vi "AM modulation_test.vi"() -> ()   [LabVIEW 2017]
uses:
  <vilib>/Analysis/baseanly.llb/Unit Vector (DBL).vi
  <vilib>/Analysis/3filter.llb/FIR Filter (DBL).vi
  <vilib>/Analysis/NI_AALBase.lvlib
  <vilib>/Analysis/NI_AALPro.lvlib
panel:
  out "ASK Modulation signal + Noise":waveform(dbl)(graph)
  out "ASK Modulation signal + Noise":waveform(dbl)(graph)
  in  "SNR(dB)":dbl=6.0
  out "불리언":bool
  out "ASK Modulation signal3":waveform(dbl)(graph)
  out "ASK Modulation signal 2":waveform(dbl)(graph)
  out "크기 2":i32
  in  "Carrier Frequency(Hz)":dbl=50000.0
  out "ASK Modulation signal":waveform(dbl)(graph)
  in  "ID":string="0110"
  out "Data Array 1":dbl[](array[numeric])
  out "Data Array 0":dbl[](array[numeric])
  in  "Data(1) time(sec)":dbl=0.1
  in  "Frequency(Hz)":dbl=30000.0
  in  "Amplitude(Vpeak)":dbl=1.0
  in  "Sampling frequency(Hz)":dbl=100000.0
  in  "Data(0) time(sec)":dbl=0.1
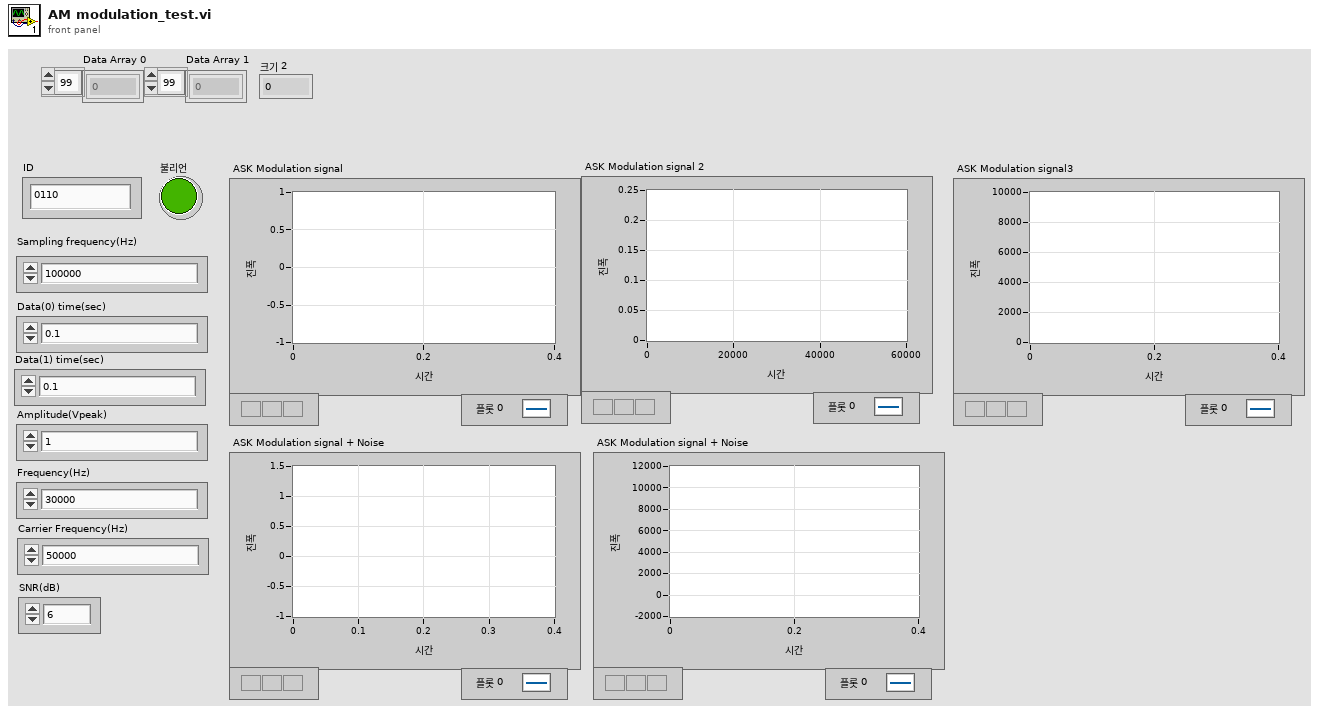
[diagram p1: front panel]
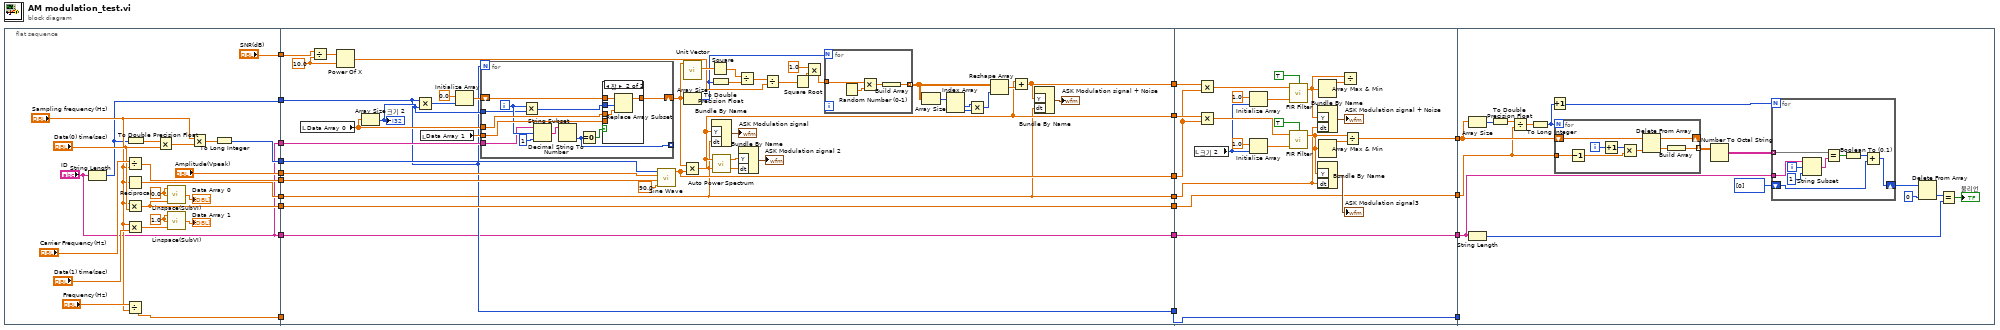
[diagram p0: block diagram]
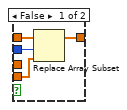
[diagram p2: hidden frame]
diagram:
  n1 = flat-sequence {
    tunnel: [w36] -> w21
    tunnel: ["Amplitude(Vpeak)"] -> w20
    tunnel: [w33] -> w19
    tunnel: [w32] -> w18
    tunnel: ["ID"] -> w17
    tunnel: [w24] -> w16
    tunnel: [w26] -> w12
    tunnel: [w25] -> w11
    tunnel: ["ID"] -> w5
    tunnel: ["SNR(dB)"] -> w2
    tunnel: w21 -> [w78]
    tunnel: w20 -> [w76]
    tunnel: w19 -> [_]
    tunnel: w18 -> [w49]
    tunnel: w17 -> [w77]
    tunnel: w16 -> [w69]
    tunnel: [w50] -> w15
    tunnel: [w72] -> w14
    tunnel: [w49] -> w13
    tunnel: w12 -> [w71]
    tunnel: w11 -> [w70]
    tunnel: [w70] -> w10
    tunnel: [w69] -> w6
    tunnel: w5 -> [w68]
    tunnel: [w68] -> w3
    tunnel: w2 -> [w67]
    tunnel: [w47] -> w1
    tunnel: w15 -> [w133]
    tunnel: w14 -> [w113]
    tunnel: w13 -> [w111]
    tunnel: w10 -> [w127]
    tunnel: [w124] -> w9
    tunnel: [w127] -> w8
    tunnel: [w123] -> w7
    tunnel: w6 -> [w123]
    tunnel: [w122] -> w4
    tunnel: w3 -> [w122]
    tunnel: w1 -> [w112]
    tunnel: w9 -> [w146]
    tunnel: w8 -> [w145]
    tunnel: w7 -> [_]
    tunnel: w4 -> [w139]
    frame #0 {
      w41 = 1.0 ("Start")
      w43 = 0.0 ("Start")
      n2 = String Length(string="ID") -> (length=w24:i32)
      n3 = Divide(x="Carrier Frequency(Hz)", y="Sampling frequency(Hz)") -> (x/y=w26:dbl)
      n4 = Reciprocal(x="Sampling frequency(Hz)") -> (1/x=w32:dbl)
      n5 = Multiply(x="Sampling frequency(Hz)", y="Data(0) time(sec)") -> (x*y=w25:dbl)
      n6 = Multiply(x="Sampling frequency(Hz)", y="Data(1) time(sec)") -> (x*y=w40:dbl)
      n7 = Divide(x="Frequency(Hz)", y="Sampling frequency(Hz)") -> (x/y=w33:dbl)
      n8 = To Double Precision Float(number=w24) -> (double precision float=w30:dbl)
      n9 = Multiply(x=w30, y="Data(0) time(sec)") -> (x*y=w29:dbl)
      n10 = call "Linspace(SubVI).vi"("NumElements"=w25, "End"=w43, "Start"=w43) -> ("Array"=→"Data Array 0":dbl[])
      n11 = call "Linspace(SubVI).vi"("NumElements"=w40, "End"=w41, "Start"=w41) -> ("Array"=→"Data Array 1":dbl[])
      n12 = Multiply(x="Sampling frequency(Hz)", y=w29) -> (x*y=w37:dbl)
      n13 = To Long Integer(number=w37) -> (32bit integer=w36:i32)
    }
    frame #1 {
      w66 = 10.0 ("y")
      n14 = local read "Data Array 0"() -> (w84:dbl[])
      n15 = Divide(x=w67, y=w66) -> (x/y=w65:dbl)
      n16 = Power Of X(1:w66, 2:w65) -> (0:w59:dbl)
      n17 = Array Size(array=w84) -> (size(s)=w82:i32)
      "크기 2" <- w82
      n18 = Multiply(x=w69, y=w82) -> (x*y=w83:i32)
      n19 = local read "Data Array 1"() -> (w86:dbl[])
      n20 = Initialize Array(0.0 ("원소"), w83) -> (w81:dbl[])
      n21 = for {
        N: w69 -> [_]
        tunnel: w84 -> [w99]
        tunnel: w86 -> [w98]
        shift-right: [w96] -> w63
        shift-left: w81 -> [w97]
        tunnel: w82 -> [w94]
        tunnel: [w92] -> _ mode=indexing
        tunnel: w77 -> [w91]
        i -> [w95]
        n22 = Multiply(x=w95, y=w94) -> (x*y=w93:i32)
        n23 = String Subset(string=w91, offset (0)=w95, length (rest)=1 ("길이(나머지)")) -> (substring=w101:string)
        n24 = Decimal String To Number(string=w101) -> (number=w92:i32)  [unwired: 2 in, 1 out]
        n25 = Equal To 0?(x=w92) -> (x = 0?=w100:bool)
        n26 = case shown="참" w100 {
          tunnel: w99 -> [_ w107]
          tunnel: w98 -> [w103 _]
          tunnel: w97 -> [w106 w110]
          tunnel: [w105 w109] -> w96
          tunnel: w93 -> [w104 w108]
          frame False {
            n27 = Replace Array Subset(array=w106, new element=w103, index=w104) -> (w105:dbl[])
          }
          frame True {
            n28 = Replace Array Subset(array=w110, new element=w107, index=w108) -> (w109:dbl[])
          }
        }
      }
      n29 = call <vilib>:"Sine Wave.vi"("samples"=w78, "amplitude"=w76, "frequency"=w71, "phase in"=90.0) -> ("sine wave"=w72:dbl[])  [unwired: 1 in, 2 out]
      n30 = call-poly <vilib>:"Unit Vector.vi"("Input Vector"=w63) -> ("norm"=w64:dbl)  [unwired: 8 in, 2 out]
      n31 = Array Size(array=w63) -> (size(s)=w57:i32)
      n32 = Multiply(x=w63, y=w72) -> (x*y=w50:dbl[])
      n33 = Square(x=w64) -> (x^2=w62:dbl)
      n34 = Bundle By Name("Y"=w50, "dt"=w49) -> (→"ASK Modulation signal":waveform(dbl))  [unwired: 1 in]
      n35 = To Double Precision Float(number=w57) -> (double precision float=w61:dbl)
      n36 = call <vilib>:"Auto Power Spectrum.vi"("dt"=w49, "Signal (V)"=w50) -> ("df"=w74:dbl, "Power Spectrum (V^2 rms)"=w75:dbl[])
      n37 = Divide(x=w62, y=w61) -> (x/y=w60:dbl)
      n38 = Bundle By Name("Y"=w75, "dt"=w74) -> (→"ASK Modulation signal 2":waveform(dbl))  [unwired: 1 in]
      n39 = Divide(x=w60, y=w59) -> (x/y=w58:dbl)
      n40 = Square Root(x=w58) -> (sqrt(x)=w46:dbl)
      n41 = Multiply(x=1.0, y=w46) -> (x*y=w44:dbl)
      n42 = for {
        N: w57 -> [_]
        tunnel: w44 -> [w89]
        tunnel: [w87] -> w52 mode=indexing
        n43 = Random Number (0-1)() -> (number: 0 to 1=w90:dbl)
        n44 = Multiply(x=w89, y=w90) -> (x*y=w88:dbl)
        n45 = Build Array(w88) -> (w87:dbl[])
      }
      n46 = Array Size(array=w52) -> (size(s)=w54:i32[])
      n47 = Index Array(array=w54) -> (element #1=w56:i32, element #2=w55:i32)  [unwired: 2 in]
      n48 = Multiply(x=w56, y=w55) -> (x*y=w53:i32)
      n49 = Reshape Array(w52, w53) -> (w51:dbl[])
      n50 = Add(x=w50, y=w51) -> (x+y=w47:dbl[])
      n51 = Bundle By Name("Y"=w47, "dt"=w49) -> (→"ASK Modulation signal + Noise":waveform(dbl))  [unwired: 1 in]
    }
    frame #2 {
      n52 = local read "크기 2"() -> (w114:i32)
      n53 = Multiply(x=w112, y=w113) -> (x*y=w119:dbl[])
      n54 = Multiply(x=w133, y=w113) -> (x*y=w130:dbl[])
      n55 = Initialize Array(1.0 ("원소"), w114) -> (w120:dbl[])
      n56 = Initialize Array(1.0 ("원소"), w114) -> (w131:dbl[])
      n57 = call-poly <vilib>:"FIR Filter.vi"("init/cont (init:F)"=TRUE, "FIR Coefficients"=w120, "X"=w119) -> ("Filtered X"=w116:dbl[])  [unwired: 1 in, 1 out]
      n58 = call-poly <vilib>:"FIR Filter.vi"("init/cont (init:F)"=TRUE, "FIR Coefficients"=w131, "X"=w130) -> ("Filtered X"=w126:dbl[])  [unwired: 1 in, 1 out]
      n59 = Bundle By Name("Y"=w116, "dt"=w111) -> (→"ASK Modulation signal + Noise":waveform(dbl))  [unwired: 1 in]
      n60 = Bundle By Name("Y"=w126, "dt"=w111) -> (→"ASK Modulation signal3":waveform(dbl))  [unwired: 1 in]
      n61 = Array Max & Min(array=w116) -> (max value=w115:dbl)  [unwired: 3 out]
      n62 = Array Max & Min(array=w126) -> (max value=w125:dbl)  [unwired: 3 out]
      n63 = Divide(x=w116, y=w115) -> ()  [unwired: 1 out]
      n64 = Divide(x=w126, y=w125) -> (x/y=w124:dbl[])
    }
    frame #3 {
      n65 = Array Size(array=w146) -> (size(s)=w149:i32)
      n66 = String Length(string=w139) -> (length=w135:i32)
      n67 = To Double Precision Float(number=w149) -> (double precision float=w148:dbl)
      n68 = Divide(x=w148, y=w145) -> (x/y=w147:dbl)
      n69 = To Long Integer(number=w147) -> (32bit integer=w144:i32)
      n70 = Increment(x=w144) -> (x+1=w143:i32)
      n71 = for {
        N: w144 -> [_]
        shift-right: [w166] -> _
        shift-left: w146 -> [w167]
        tunnel: w145 -> [w165]
        tunnel: [w162] -> w141 mode=indexing
        i -> [w161]
        n72 = Decrement(x=w165) -> (x-1=w164:dbl)
        n73 = Increment(x=w161) -> (x+1=w160:i32)
        n74 = Multiply(x=w160, y=w164) -> (x*y=w163:dbl)
        n75 = Delete From Array(array=w167, index=w163) -> (deleted portion=w159:dbl, array with subset deleted=w166:dbl[])  [unwired: 1 in]
        n76 = Build Array(w159) -> (w162:dbl[])
      }
      n77 = Number To Octal String(2:w141) -> (0:w142:string[][])  [unwired: 1 in]
      n78 = for {
        N: w143 -> [_]
        tunnel: w139 -> [w158]
        tunnel: w142 -> [w156] mode=indexing
        shift-right: [w150] -> w138
        shift-left: i32[] [0] -> [w151]
        i -> [w157]
        n79 = String Subset(string=w158, offset (0)=w157, length (rest)=1 ("길이(나머지)")) -> (substring=w154:string)
        n80 = Equal?(x=w156, y=w154) -> (x = y?=w153:bool[])
        n81 = Boolean To (0,1)(Boolean=w153) -> (0, 1=w152:i16[])
        n82 = Add(x=w152, y=w151) -> (x+y=w150:i32[])
      }
      n83 = Delete From Array(array=w138, index=0 ("인덱스")) -> (deleted portion=w136:i32)  [unwired: 1 in, 1 out]
      n84 = Equal?(x=w136, y=w135) -> (x = y?=→"불리언":bool)
    }
  }
